vi "Configure Noise.vi"(5 "BandWidth (80 MHz)":dbl=80000000.0 format="%#.3g", 6 "Standard Deviation (0.008 V)":dbl=0.008 format="%#.4g", 7 "Enable BandSet (T:Enable)":bool=TRUE, 8 "error in (no error)":errorcluster, 9 "Mean (0.00 V)":dbl min=-9.996 max=9.996 format="%#.3g", 10 "Channel (1:Channel 1)":i32(ring)=1 items=["Channel 1"=1, "Channel 2"=2], 11 "VISA resource name":refnum<visa-resource-name>) -> (0 "error out":errorcluster, 3 "VISA resource name out":refnum<visa-resource-name>)   [LabVIEW 2015, in "SDG X Series.lvlib"]
doc: "Configures Noise waveform and parameters."
uses:
  <instrlib>/SDG X Series/SDG X Series.lvlib
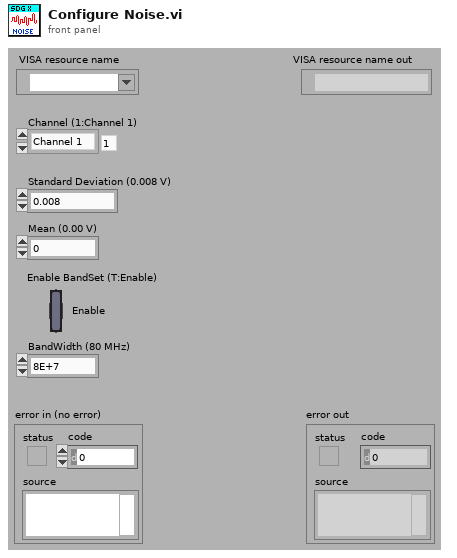
[diagram p1: front panel]
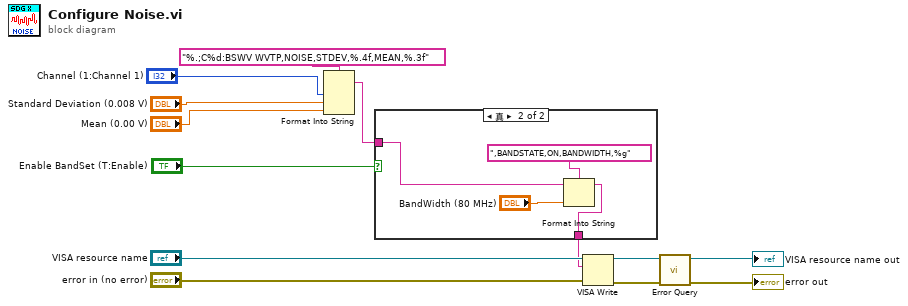
[diagram p0: block diagram]
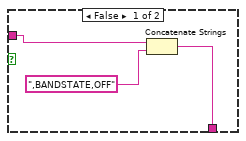
[diagram p2: hidden frame]
diagram:
  n1 = Format Into String(format string="%.;C%d:BSWV WVTP,NOISE,STDEV,%.4f,MEAN,%.3f", "Channel (1:Channel 1)", "Standard Deviation (0.008 V)", "Mean (0.00 V)") -> (resulting string=w3:string)  [unwired: 2 in, 1 out]
  n2 = case shown="真" "Enable BandSet (T:Enable)" {
    tunnel: w3 -> [w16 w18]
    tunnel: [w14 w17] -> w2
    frame False {
      n3 = Concatenate Strings(w16, ",BANDSTATE,OFF" ("格式字符串")) -> (w14:string)
    }
    frame True {
      n4 = Format Into String(format string=",BANDSTATE,ON,BANDWIDTH,%g" ("格式字符串"), initial string=w18, "BandWidth (80 MHz)") -> (resulting string=w17:string)  [unwired: 1 in, 1 out]
    }
  }
  n5 = VISA Write(VISA resource name="VISA resource name", write buffer=w2, error in (no error)="error in (no error)") -> (VISA resource name out=w11:refnum<visa-resource-name>, error out=w10:errorcluster)  [unwired: 1 out]
  n6 = call <instrlib>:"Error Query.vi"("error in (no error)"=w10, "VISA resource name"=w11) -> ("error out"=→"error out":errorcluster, "VISA resource name out"=→"VISA resource name out":refnum<visa-resource-name>)  [unwired: 6 in, 2 out]
